vi "Limelight.vi"() -> (5 "value":T1)   [LabVIEW 2023]
uses:
  <vilib>/Rock Robotics/Network Tables/NT Read Numeric Array.vi
  <vilib>/Analysis/NI_AALBase.lvlib
  <vilib>/Analysis/baseanly.llb/Mean (DBL).vi
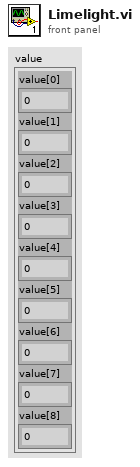
[diagram p1: front panel]
types:
  T1 = cluster{"value[0]":dbl, "value[1]":dbl, "value[2]":dbl, "value[3]":dbl, "value[4]":dbl, "value[5]":dbl, "value[6]":dbl, "value[7]":dbl, "value[8]":dbl}
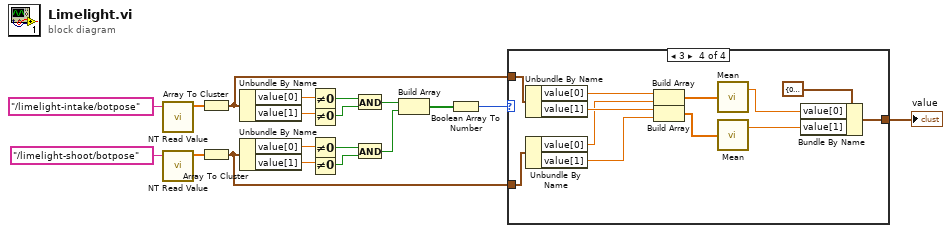
[diagram p0: block diagram]
diagram:
  n1 = call-poly <vilib>:"NT Read Value.vi"("name"="/limelight-intake/botpose" ("Name")) -> ("value"=w19:dbl[])  [unwired: 8 in, 2 out]
  n2 = call-poly <vilib>:"NT Read Value.vi"("name"="/limelight-shoot/botpose" ("Name")) -> ("value"=w8:dbl[])  [unwired: 8 in, 2 out]
  n3 = Array To Cluster(array=w19) -> (cluster=w2:T1)
  n4 = Array To Cluster(array=w8) -> (cluster=w1:T1)
  n5 = Unbundle By Name(w2) -> ("value[0]"=w17:dbl, "value[1]"=w16:dbl)
  n6 = Unbundle By Name(w1) -> ("value[0]"=w10:dbl, "value[1]"=w11:dbl)
  n7 = Not Equal To 0?(x=w17) -> (x != 0?=w14:bool)
  n8 = Not Equal To 0?(x=w16) -> (x != 0?=w15:bool)
  n9 = Not Equal To 0?(x=w10) -> (x != 0?=w13:bool)
  n10 = Not Equal To 0?(x=w11) -> (x != 0?=w12:bool)
  n11 = And(x=w14, y=w15) -> (x .and. y?=w7:bool)
  n12 = And(x=w13, y=w12) -> (x .and. y?=w6:bool)
  n13 = Build Array(w7, w6) -> (w5:bool[])
  n14 = Boolean Array To Number(Boolean array=w5) -> (number=w4:u32)
  n15 = case shown="3" w4 {
    tunnel: [_ w20 w21 w22] -> w3
    tunnel: w2 -> [_ w20 _ w33]
    tunnel: w1 -> [_ _ w21 w32]
    frame 0, Default {
    }
    frame 1 {
    }
    frame 2 {
    }
    frame 3 {
      n16 = Unbundle By Name(w33) -> ("value[0]"=w31:dbl, "value[1]"=w30:dbl)
      n17 = Unbundle By Name(w32) -> ("value[0]"=w29:dbl, "value[1]"=w28:dbl)
      n18 = Build Array(w31, w29) -> (w27:dbl[])
      n19 = Build Array(w30, w28) -> (w26:dbl[])
      n20 = call-poly <vilib>:"Mean.vi"("X"=w27) -> ("mean"=w24:dbl)  [unwired: 1 out]
      n21 = call-poly <vilib>:"Mean.vi"("X"=w26) -> ("mean"=w23:dbl)  [unwired: 1 out]
      n22 = Bundle By Name(cluster=T1 {"value[0]"=0.0, "value[1]"=0.0, "value[2]"=0.0, "value[3]"=0.0, "value[4]"=0.0, "value[5]"=0.0, "value[6]"=0.0, "value[7]"=0.0, "value[8]"=0.0} ("value"), "value[0]"=w24, "value[1]"=w23) -> (w22:T1)
    }
  }
  "value" <- w3
